vi "Engine-DI-Host.vi"() -> ()   [LabVIEW 2016]
uses:
  <vilib>/addons/Software Calibration Management/XControls/TBL2D.xctl
  <vilib>/Utility/miscctls.llb/LVRowAndColumnTypeDef.ctl
panel:
  in  "_Refresh PW Table":bool
  in  "_Hidden":enum32{"Page 1"}(tab)
  in  "InjQtys_Man":sgl[][](array[numeric]) caption="[]"
  in  "InjSplits":sgl[][](array[numeric]) caption="[]"
  out "CylFuelQtys":sgl[](array[numeric]) caption="[mm3/cycle/cyl]"
  in  "CylSplits":sgl[](array[numeric]) caption="[%]"
  out "InjQtys":sgl[][](array[numeric]) caption="[]"
  in  "_Refresh Table":bool
  out "Channels|Names":string[](array[string])
  out "Pulsewidths":sgl[][](array[numeric]) caption="[]"
  in  "_Bank Selection":T1(tab)
  out "TotalFuelQty":sgl caption="[mm3/cyc]"
  out "_Total Fueling Rate":sgl(graph) caption="[mm3/cyc]"
  in  "_Cylinder Fueling Control":i32(listbox) caption="DI Fueling Quantities"
  in  "InjQtys_ManE":bool caption="Mode Select"
  in  "_Cyl Split":sgl caption="Cylinder Split [%]"
  in  "_InjSplits":sgl[](array[numeric]) caption="Injection Splits [%]"
  in  "_InjQtys_Man":sgl[](array[numeric]) caption="Manual Injection Quantities [mm3/inj]"
  out "_Total Fueling Rate Indicator":sgl caption="[mm3/cyc]"
  in  "Enable":bool caption="Control Mode"
  in  "MinInjPW_A":sgl caption="[ms]"
  in  "InjFlowCal_A":cluster{"X":sgl[], "Y":sgl[], "Z":sgl[][]}(xcontrol) caption="[%|RPM|mm3/stroke]"
  in  "DI-A_RailPIndex":i32(ring) items=["None"=-1, "AI01"=0, "AI02"=1, "AI03"=2, "AI04"=3, "AI05"=4, "AI06"=5, "AI07"=6, "AI08"=7, "AI09"=8, "AI10"=9, "AI11"=10, "AI12"=11]
  out "DI-A_RailPSensor":T2 {"Value" format="%#_4p"}
  in  "MinInjPW_B":sgl caption="[ms]"
  in  "InjFlowCal_B":cluster{"X":sgl[], "Y":sgl[], "Z":sgl[][]}(xcontrol) caption="[%|RPM|mm3/stroke]"
  in  "DI-B_RailPIndex":i32(ring) items=["None"=-1, "AI01"=0, "AI02"=1, "AI03"=2, "AI04"=3, "AI05"=4, "AI06"=5, "AI07"=6, "AI08"=7, "AI09"=8, "AI10"=9, "AI11"=10, "AI12"=11]
  out "DI-B_RailPSensor":T2 {"Value" format="%#_4p"}
  in  "_Pulsewidths":i32(listbox) caption="DI Pulsewidths"
  # "DI Control and Calibration"
  # "Total DI Fueling Rate"
  # "RailP Sensor"
  # "Value"
  # "Units"
  # "RailP Sensor"
  # "Value"
  # "Units"
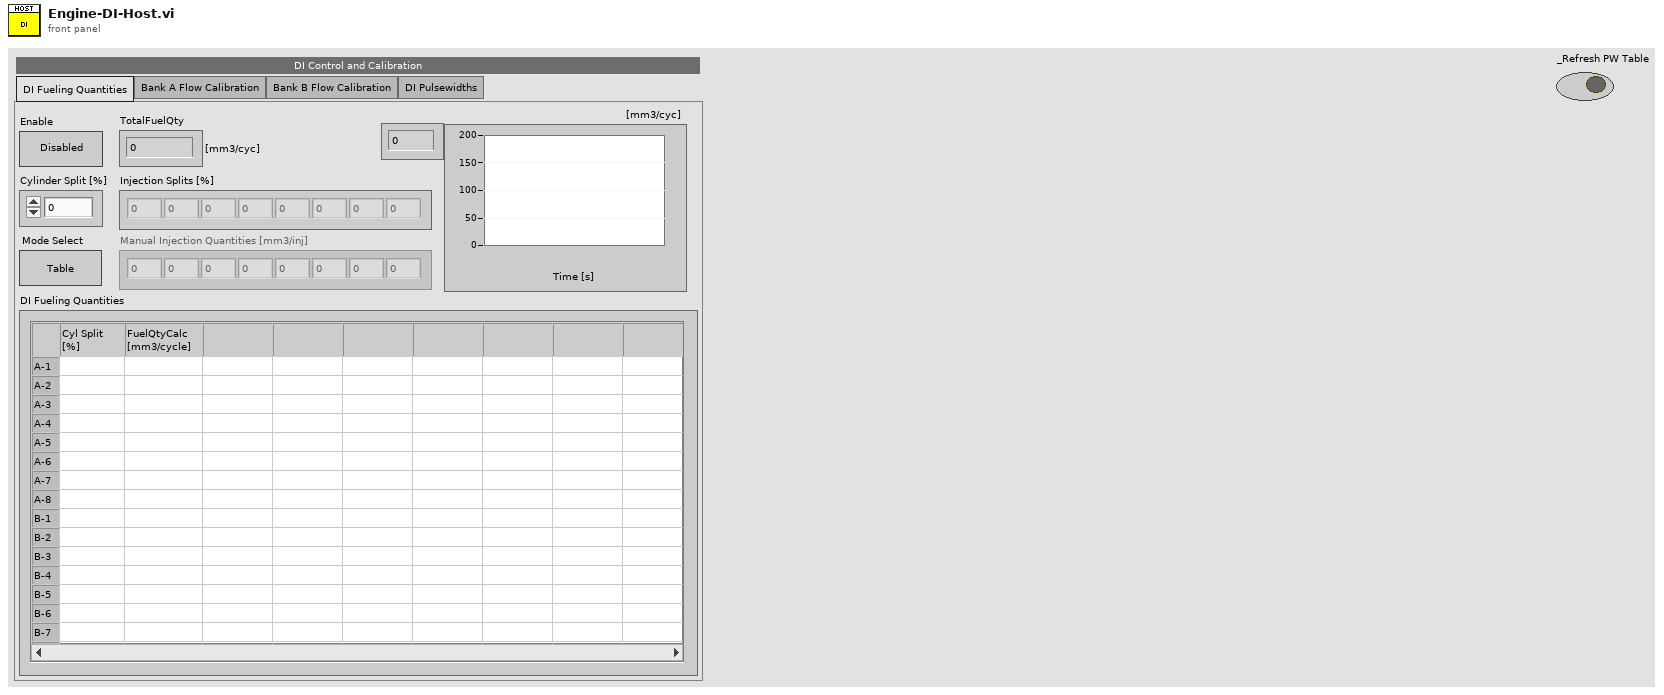
[diagram p1: front panel]
types:
  T1 = enum32{"DI Fueling Quantities", "Bank A Flow Calibration", "Bank B Flow Calibration", "DI Pulsewidths"}
  T2 = cluster{"Name":string, "Unit":string, "Value":sgl}
  T3 = typedef "LVRowAndColumnTypeDef.ctl" = cluster{"Row":i32, "Column":i32}
  T4 = enum8{"Enabled", "Disabled", "Disabled and Grayed Out"}
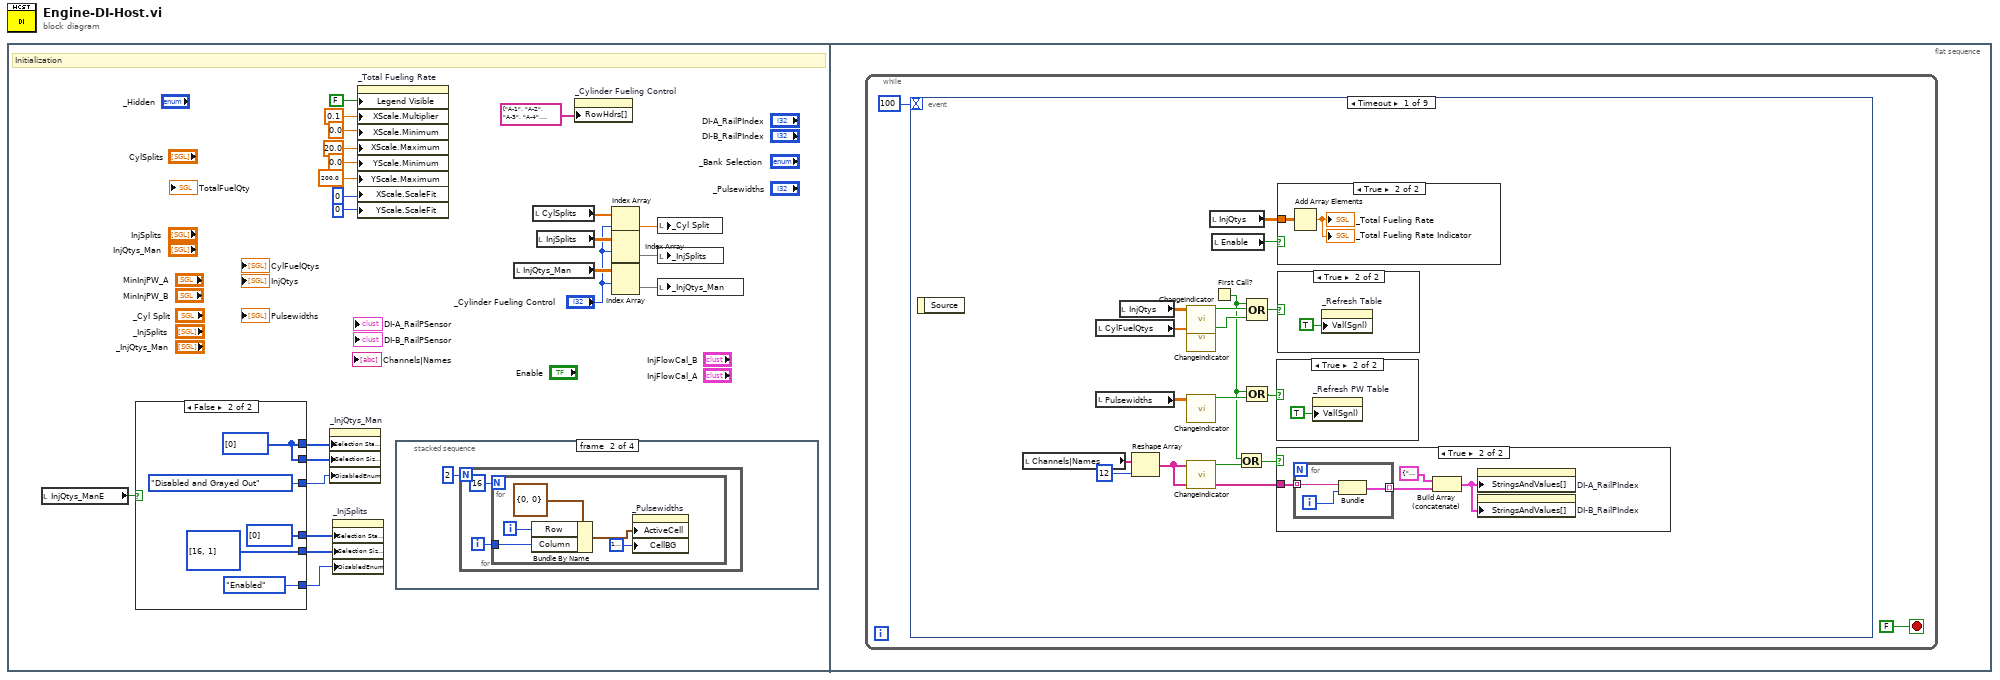
[diagram p0: block diagram]
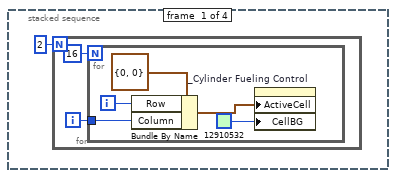
[diagram p2: hidden frame]
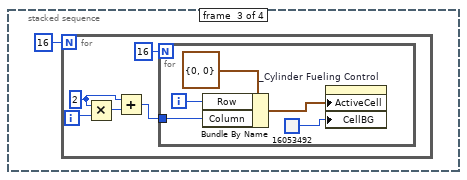
[diagram p3: hidden frame]
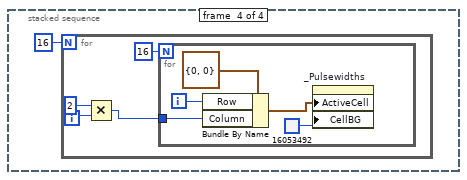
[diagram p4: hidden frame]
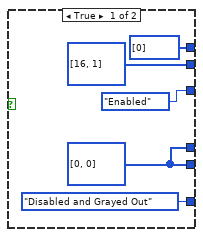
[diagram p5: hidden frame]
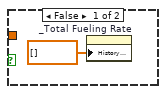
[diagram p9: hidden frame]
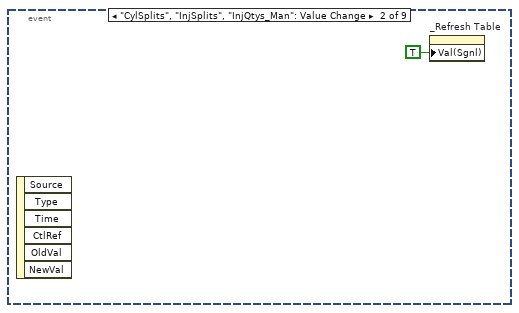
[diagram p10: hidden frame]
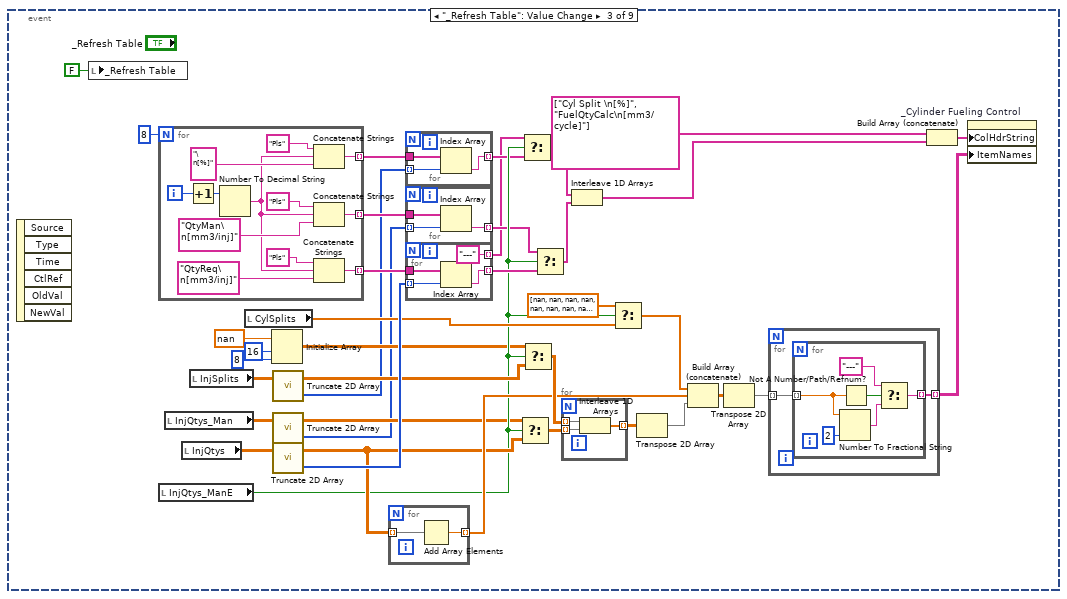
[diagram p11: hidden frame]
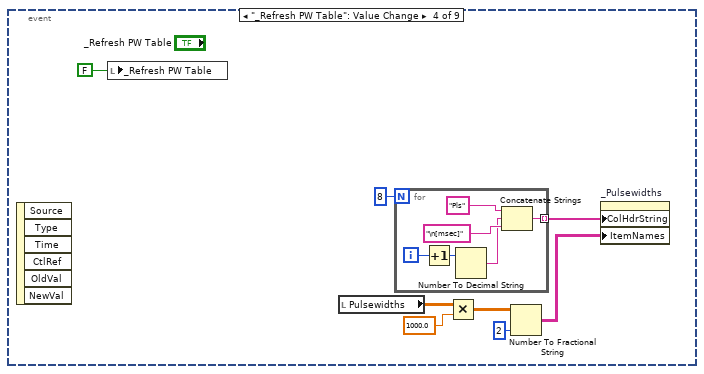
[diagram p12: hidden frame]
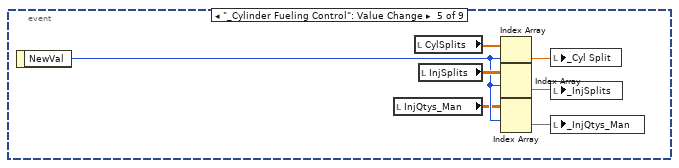
[diagram p13: hidden frame]
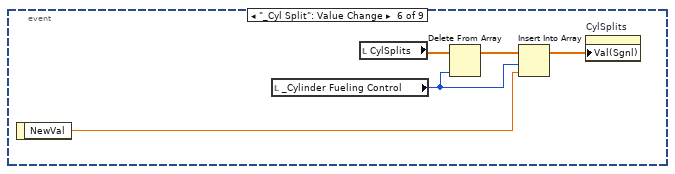
[diagram p14: hidden frame]
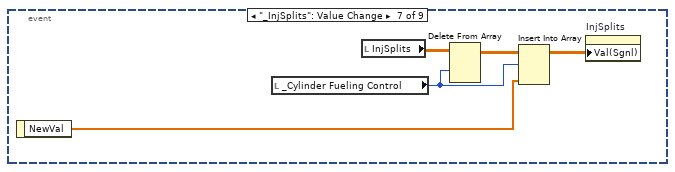
[diagram p15: hidden frame]
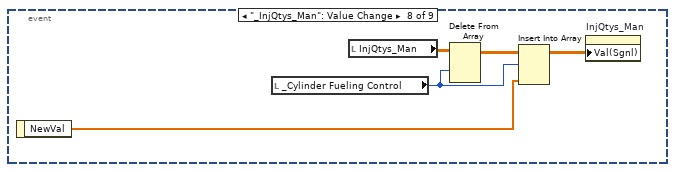
[diagram p16: hidden frame]
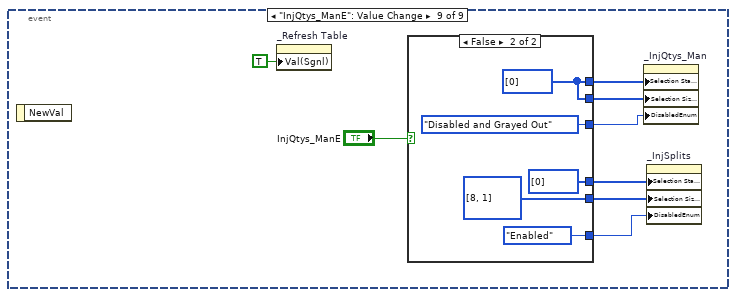
[diagram p17: hidden frame]
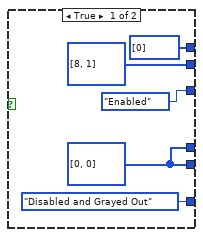
[diagram p18: hidden frame]
diagram:
  n1 = flat-sequence {
    frame #0 {
      # "Initialization"
      n2 = local read "InjQtys_ManE"() -> (w1:bool)
      n3 = case shown="False" w1 {
        tunnel: [u32[] [16, 1] ("Selection Start[]") w68] -> w7
        tunnel: [w63 u32[] [16, 1] ("Selection Start[]")] -> w6
        tunnel: [u32[] [0] ("Selection Size[]") w68] -> w5
        tunnel: [w63 u32[] [0] ("Selection Size[]")] -> w4
        tunnel: [T4."Enabled" ("Disabled") T4."Disabled and Grayed Out" ("Disabled")] -> w3
        tunnel: [T4."Disabled and Grayed Out" ("Disabled") T4."Enabled" ("Disabled")] -> w2
        frame True {
          w63 = u32[] [0, 0] ("Selection Start[]")
        }
        frame False {
          w68 = u32[] [0] ("Selection Size[]")
        }
      }
      n4 = property on="_InjQtys_Man" class="Arr (strict)"("Selection Start []"=w5, "Selection Size []"=w7, "DisabledEnum"=w3) -> ()  [unwired: 2 in, 2 out]
      n5 = property on="_InjSplits" class="Arr (strict)"("Selection Start []"=w4, "Selection Size []"=w6, "DisabledEnum"=w2) -> ()  [unwired: 2 in, 2 out]
      n6 = property on="_Total Fueling Rate" class="WFChart (strict)"("Legend Visible"=FALSE ("Legend:Visible"), "XScale.Multiplier"=0.1 ("X Scale.Range:Maximum"), "XScale.Minimum"=0.0 ("X Scale.Range:Minimum"), "XScale.Maximum"=20.0 ("X Scale.Range:Maximum"), "YScale.Minimum"=0.0 ("Y Scale.Range:Minimum"), "YScale.Maximum"=200.0 ("Y Scale.Range:Maximum"), "XScale.ScaleFit"=u8 0 ("X Scale.Scale Fit"), "YScale.ScaleFit"=u8 0 ("Y Scale.Scale Fit")) -> ()  [unwired: 2 in, 2 out]
      n7 = stacked-sequence {
        frame #0 {
          n8 = for {
            N: 2 -> [_]
            i -> [w25]
            n9 = for {
              N: 16 -> [_]
              tunnel: w25 -> [w27]
              i -> [w30]
              n10 = Bundle By Name(cluster=T3 {"Row"=0, "Column"=0} ("Active Cell:Active Cell"), "Row"=w30, "Column"=w27) -> (w29:T3)
              n11 = property on="_Cylinder Fueling Control" class="MCListbox (strict)"("ActiveCell"=w29, "CellBG"=u32 12910532) -> ()  [unwired: 2 in, 2 out]
            }
          }
        }
        frame #1 {
          n12 = for {
            N: 2 -> [_]
            i -> [w33]
            n13 = for {
              N: 16 -> [_]
              tunnel: w33 -> [w35]
              i -> [w38]
              n14 = Bundle By Name(cluster=T3 {"Row"=0, "Column"=0} ("Active Cell:Active Cell"), "Row"=w38, "Column"=w35) -> (w37:T3)
              n15 = property on="_Pulsewidths" class="MCListbox (strict)"("ActiveCell"=w37, "CellBG"=u32 16777226) -> ()  [unwired: 2 in, 2 out]
            }
          }
        }
        frame #2 {
          n16 = for {
            N: 16 -> [_]
            i -> [w44]
            w41 = 2
            n17 = Multiply(x=w41, y=w44) -> (x*y=w43:i32)
            n18 = Add(x=w41, y=w43) -> (x+y=w42:i32)
            n19 = for {
              N: 16 -> [_]
              tunnel: w42 -> [w47]
              i -> [w49]
              n20 = Bundle By Name(cluster=T3 {"Row"=0, "Column"=0} ("Active Cell:Active Cell"), "Row"=w49, "Column"=w47) -> (w48:T3)
              n21 = property on="_Cylinder Fueling Control" class="MCListbox (strict)"("ActiveCell"=w48, "CellBG"=u32 16053492) -> ()  [unwired: 2 in, 2 out]
            }
          }
        }
        frame #3 {
          n22 = for {
            N: 16 -> [_]
            i -> [w54]
            n23 = Multiply(x=2, y=w54) -> (x*y=w52:i32)
            n24 = for {
              N: 16 -> [_]
              tunnel: w52 -> [w57]
              i -> [w59]
              n25 = Bundle By Name(cluster=T3 {"Row"=0, "Column"=0} ("Active Cell:Active Cell"), "Row"=w59, "Column"=w57) -> (w58:T3)
              n26 = property on="_Pulsewidths" class="MCListbox (strict)"("ActiveCell"=w58, "CellBG"=u32 16053492) -> ()  [unwired: 2 in, 2 out]
            }
          }
        }
      }
      n27 = local read "InjQtys_Man"() -> (w22:sgl[][])
      n28 = local read "CylSplits"() -> (w18:sgl[])
      n29 = local read "InjSplits"() -> (w20:sgl[][])
      n30 = property on="_Cylinder Fueling Control" class="MCListbox (strict)"("RowHdrs[]"=string[] ["A-1", "A-2", "A-3", "A-4", "A-5", "A-6", "A-7", "A-8", "B-1", "B-2", "B-3", "B-4", "B-5", "B-6", "B-7", "B-8"] ("Row Header Strings[]")) -> ()  [unwired: 2 in, 2 out]
      n31 = Index Array(array=w18, index="_Cylinder Fueling Control") -> (element=w19:sgl)
      n32 = Index Array(array=w20, index (row)="_Cylinder Fueling Control") -> (element=w21:sgl[])  [unwired: 1 in]
      n33 = Index Array(array=w22, index (row)="_Cylinder Fueling Control") -> (element=w23:sgl[])  [unwired: 1 in]
      n34 = local write "_Cyl Split"(w19) -> ()
      n35 = local write "_InjSplits"(w21) -> ()
      n36 = local write "_InjQtys_Man"(w23) -> ()
    }
    frame #1 {
      n37 = while {
        stop <- FALSE stop-if-true
        n38 = event shown="[0] Timeout" {
          selector: _ -> [_ _ _ _ _ _ _ _ _]
          dyn-events: _ -> [_ _ _ _ _ _ _ _ _]
          timeout: 100 -> [_ _ _ _ _ _ _ _ _]
          event Timeout {
            n39 = event-data() -> ()  [unwired: 1 in, 1 out]
            n40 = local read "Channels|Names"() -> (w75:string[])
            n41 = local read "CylFuelQtys"() -> (w86:sgl[])
            n42 = local read "Pulsewidths"() -> (w81:sgl[][])
            n43 = local read "InjQtys"() -> (w85:sgl[][])
            n44 = Reshape Array(w75, 12 ("dimension size")) -> (w73:string[])
            n45 = call "ChangeIndicator.vi"("Input"=w85) -> ("Change"=w83:bool)  [unwired: 9 in]
            n46 = call "ChangeIndicator.vi"("Input"=w86) -> ("Change"=w84:bool)  [unwired: 9 in]
            n47 = call "ChangeIndicator.vi"("Input"=w81) -> ("Change"=w79:bool)  [unwired: 9 in]
            n48 = call "ChangeIndicator.vi"("Input"=w73) -> ("Change"=w77:bool)  [unwired: 9 in]
            n49 = local read "InjQtys"() -> (w87:sgl[][])
            n50 = First Call?() -> (First Call?: T/F=w78:bool)
            n51 = local read "Enable"() -> (w88:bool)
            n52 = Or(x=w78, y=w77) -> (x .or. y?=w76:bool)
            n53 = Compound Arithmetic op=OR(w78, w83, w84) -> (w82:bool)
            n54 = Compound Arithmetic op=OR(w78, w79) -> (w80:bool)
            n55 = case shown="True" w80 {
              frame False {
              }
              frame True {
                n56 = property on="_Refresh PW Table" class="Bool (strict)"("Val(Sgnl)"=TRUE ("Value (Signaling)")) -> ()  [unwired: 2 in, 2 out]
              }
            }
            n57 = case shown="True" w76 {
              tunnel: w73 -> [_ w92]
              frame False {
              }
              frame True {
                n58 = for {
                  tunnel: w92 -> [w95] mode=indexing
                  tunnel: [w93] -> w91 mode=indexing
                  i -> [w94]
                  n59 = Bundle("String"=w95, w94) -> (w93:cluster{"String":string, i32})  [unwired: 1 in]
                }
                n60 = Build Array (concatenate)(cluster{"String":string, i32} {"String"="None", -1} ("cluster"), w91) -> (w90:cluster{"String":string, i32}[])
                n61 = property on="DI-A_RailPIndex" class="Ring (strict)"("StringsAndValues[]"=w90) -> ()  [unwired: 2 in, 2 out]
                n62 = property on="DI-B_RailPIndex" class="Ring (strict)"("StringsAndValues[]"=w90) -> ()  [unwired: 2 in, 2 out]
              }
            }
            n63 = case shown="True" w88 {
              tunnel: w87 -> [_ w100]
              frame False {
                n64 = property on="_Total Fueling Rate" class="WFChart (strict)"("History Data"=sgl[] []) -> ()  [unwired: 2 in, 2 out]
              }
              frame True {
                n65 = Add Array Elements(numeric array=w100) -> (sum=→"_Total Fueling Rate" →"_Total Fueling Rate Indicator":sgl)
              }
            }
            n66 = case shown="True" w82 {
              frame False {
              }
              frame True {
                n67 = property on="_Refresh Table" class="Bool (strict)"("Val(Sgnl)"=TRUE ("Value (Signaling)")) -> ()  [unwired: 2 in, 2 out]
              }
            }
          }
          event "CylSplits", "InjSplits", "InjQtys_Man": Value Change {
            n68 = event-data() -> ()  [unwired: 1 in, 6 out]
            n69 = property on="_Refresh Table" class="Bool (strict)"("Val(Sgnl)"=TRUE ("Value (Signaling)")) -> ()  [unwired: 2 in, 2 out]
          }
          event "_Refresh Table": Value Change {
            n70 = event-data() -> ()  [unwired: 1 in, 6 out]
            n71 = local write "_Refresh Table"(FALSE ("_Refresh Table")) -> ()
            n72 = for {
              N: 8 -> [_]
              tunnel: [w172] -> w138 mode=indexing
              tunnel: [w168] -> w137 mode=indexing
              tunnel: [w164] -> w139 mode=indexing
              i -> [w175]
              n73 = Increment(x=w175) -> (x+1=w174:i32)
              n74 = Number To Decimal String(number=w174) -> (decimal integer string=w166:string)  [unwired: 1 in]
              n75 = Concatenate Strings("Pls", w166, "\n[%]") -> (w168:string)
              n76 = Concatenate Strings("Pls", w166, "QtyMan\n[mm3/inj]") -> (w172:string)
              n77 = Concatenate Strings("Pls", w166, "QtyReq\n[mm3/inj]") -> (w164:string)
            }
            n78 = local read "InjQtys_ManE"() -> (w109:bool)
            n79 = local read "InjQtys_Man"() -> (w130:sgl[][])
            n80 = local read "InjQtys"() -> (w129:sgl[][])
            n81 = local read "InjSplits"() -> (w131:sgl[][])
            n82 = local read "CylSplits"() -> (w127:sgl[])
            n83 = Initialize Array(sgl nan ("Numeric"), 16 ("dimension size"), 8 ("dimension size")) -> (w107:sgl[][])
            n84 = call "Truncate 2D Array.vi"("2D Array"=w131) -> ("Header Index"=w104:i32[], "Truncated 2D Array"=w136:sgl[][])  [unwired: 1 in]
            n85 = call "Truncate 2D Array.vi"("2D Array"=w130) -> ("Header Index"=w103:i32[], "Truncated 2D Array"=w108:sgl[][])  [unwired: 1 in]
            n86 = call "Truncate 2D Array.vi"("2D Array"=w129) -> ("Header Index"=w140:i32[], "Truncated 2D Array"=w113:sgl[][])  [unwired: 1 in]
            n87 = for {
              tunnel: w113 -> [w142] mode=indexing
              tunnel: [w141] -> w117 mode=indexing
              n88 = Add Array Elements(numeric array=w142) -> (sum=w141:sgl)
            }
            n89 = for {
              tunnel: w137 -> [w163]
              tunnel: w104 -> [w162] mode=indexing
              tunnel: [w161] -> w105 mode=indexing
              # "i"
              n90 = Index Array(array=w163, index=w162) -> (element=w161:string)
            }
            n91 = for {
              tunnel: w138 -> [w160]
              tunnel: w103 -> [w159] mode=indexing
              tunnel: [w158] -> w106 mode=indexing
              # "i"
              n92 = Index Array(array=w160, index=w159) -> (element=w158:string)
            }
            n93 = for {
              tunnel: w139 -> [w157]
              tunnel: w140 -> [w156] mode=indexing
              tunnel: [w155] -> w111 mode=indexing
              tunnel: ["---"] -> w102 mode=indexing
              # "i"
              n94 = Index Array(array=w157, index=w156) -> (element=w155:string)
            }
            n95 = Select(t=w108, s=w109, f=w113) -> (s? t:f=w112:sgl[][])
            n96 = Select(t=w102, s=w109, f=w105) -> (s? t:f=w120:string[])
            n97 = Select(t=w107, s=w109, f=w136) -> (s? t:f=w123:sgl[][])
            n98 = Select(t=w106, s=w109, f=w111) -> (s? t:f=w110:string[])
            n99 = for {
              tunnel: w123 -> [w145] mode=indexing
              tunnel: [w144] -> w122 mode=indexing
              tunnel: w112 -> [w143] mode=indexing
              n100 = Interleave 1D Arrays(w145, w143) -> (w144:sgl[])
            }
            n101 = Interleave 1D Arrays(w120, w110) -> (w119:string[])
            n102 = Select(t=sgl[] [nan, nan, nan, nan, nan, nan, nan, nan, nan, nan, nan, nan, nan, nan, nan, nan], s=w109, f=w127) -> (s? t:f=w126:sgl[])
            n103 = Transpose 2D Array(2D array=w122) -> (transposed array=w121:sgl[][])
            n104 = Build Array (concatenate)(w126, w117, w121) -> (w135:sgl[][])
            n105 = Transpose 2D Array(2D array=w135) -> (transposed array=w124:sgl[][])
            n106 = for {
              tunnel: w124 -> [w147] mode=indexing
              tunnel: [w146] -> w125 mode=indexing
              n107 = for {
                tunnel: w147 -> [w150] mode=indexing
                tunnel: [w148] -> w146 mode=indexing
                n108 = Number To Fractional String(number=w150, precision (6)=i16 2) -> (F-format string=w149:string)  [unwired: 2 in]
                n109 = Not A Number/Path/Refnum?(number/path/refnum=w150) -> (NaN/Path/Refnum?=w153:bool)
                n110 = Select(t="---", s=w153, f=w149) -> (s? t:f=w148:string)
              }
            }
            n111 = Build Array (concatenate)(string[] ["Cyl Split \n[%]", "FuelQtyCalc\n[mm3/cycle]"] ("Column Header Strings[]"), w119) -> (w134:string[])
            n112 = property on="_Cylinder Fueling Control" class="MCListbox (strict)"("ColHdrString"=w134, "ItemNames"=w125) -> ()  [unwired: 2 in, 2 out]
          }
          event "_Refresh PW Table": Value Change {
            n113 = event-data() -> ()  [unwired: 1 in, 6 out]
            n114 = local write "_Refresh PW Table"(FALSE ("_Refresh Table")) -> ()
            n115 = local read "Pulsewidths"() -> (w177:sgl[][])
            n116 = for {
              N: 8 -> [_]
              tunnel: [w185] -> w179 mode=indexing
              i -> [w189]
              n117 = Increment(x=w189) -> (x+1=w188:i32)
              n118 = Number To Decimal String(number=w188) -> (decimal integer string=w184:string)  [unwired: 1 in]
              n119 = Concatenate Strings("Pls", w184, "\n[msec]") -> (w185:string)
            }
            n120 = Multiply(x=w177, y=sgl 1000.0) -> (x*y=w178:sgl[][])
            n121 = Number To Fractional String(number=w178, precision (6)=i16 2) -> (F-format string=w180:string[][])  [unwired: 2 in]
            n122 = property on="_Pulsewidths" class="MCListbox (strict)"("ColHdrString"=w179, "ItemNames"=w180) -> ()  [unwired: 2 in, 2 out]
          }
          event "_Cylinder Fueling Control": Value Change {
            n123 = event-data() -> ("NewVal"=w192:i32)  [unwired: 1 in]
            n124 = local read "InjQtys_Man"() -> (w191:sgl[][])
            n125 = local read "CylSplits"() -> (w196:sgl[])
            n126 = local read "InjSplits"() -> (w194:sgl[][])
            n127 = Index Array(array=w196, index=w192) -> (element=w195:sgl)
            n128 = Index Array(array=w194, index (row)=w192) -> (element=w193:sgl[])  [unwired: 1 in]
            n129 = Index Array(array=w191, index (row)=w192) -> (element=w190:sgl[])  [unwired: 1 in]
            n130 = local write "_Cyl Split"(w195) -> ()
            n131 = local write "_InjSplits"(w193) -> ()
            n132 = local write "_InjQtys_Man"(w190) -> ()
          }
          event "_Cyl Split": Value Change {
            n133 = event-data() -> ("NewVal"=w197:sgl)  [unwired: 1 in]
            n134 = local read "_Cylinder Fueling Control"() -> (w201:i32)
            n135 = local read "CylSplits"() -> (w200:sgl[])
            n136 = Delete From Array(array=w200, index=w201) -> (array with subset deleted=w198:sgl[])  [unwired: 1 in, 1 out]
            n137 = Insert Into Array(array=w198, index=w201, new element=w197) -> (w199:sgl[])
            n138 = property on="CylSplits" class="Arr (strict)"("Val(Sgnl)"=w199) -> ()  [unwired: 2 in, 2 out]
          }
          event "_InjSplits": Value Change {
            n139 = event-data() -> ("NewVal"=w202:sgl[])  [unwired: 1 in]
            n140 = local read "_Cylinder Fueling Control"() -> (w206:i32)
            n141 = local read "InjSplits"() -> (w205:sgl[][])
            n142 = Delete From Array(array=w205, index (row)=w206) -> (array with subset deleted=w203:sgl[][])  [unwired: 2 in, 1 out]
            n143 = Insert Into Array(array=w203, index (row)=w206, new element=w202) -> (w204:sgl[][])  [unwired: 1 in]
            n144 = property on="InjSplits" class="Arr (strict)"("Val(Sgnl)"=w204) -> ()  [unwired: 2 in, 2 out]
          }
          event "_InjQtys_Man": Value Change {
            n145 = event-data() -> ("NewVal"=w207:sgl[])  [unwired: 1 in]
            n146 = local read "_Cylinder Fueling Control"() -> (w211:i32)
            n147 = local read "InjQtys_Man"() -> (w210:sgl[][])
            n148 = Delete From Array(array=w210, index (row)=w211) -> (array with subset deleted=w208:sgl[][])  [unwired: 2 in, 1 out]
            n149 = Insert Into Array(array=w208, index (row)=w211, new element=w207) -> (w209:sgl[][])  [unwired: 1 in]
            n150 = property on="InjQtys_Man" class="Arr (strict)"("Val(Sgnl)"=w209) -> ()  [unwired: 2 in, 2 out]
          }
          event "InjQtys_ManE": Value Change {
            n151 = event-data() -> ()  [unwired: 1 in, 1 out]
            n152 = property on="_Refresh Table" class="Bool (strict)"("Val(Sgnl)"=TRUE ("Value (Signaling)")) -> ()  [unwired: 2 in, 2 out]
            n153 = case shown="False" "InjQtys_ManE" {
              tunnel: [u32[] [8, 1] ("Selection Start[]") w227] -> w219
              tunnel: [w222 u32[] [8, 1] ("Selection Start[]")] -> w218
              tunnel: [u32[] [0] ("Selection Size[]") w227] -> w216
              tunnel: [w222 u32[] [0] ("Selection Size[]")] -> w215
              tunnel: [T4."Enabled" ("Disabled") T4."Disabled and Grayed Out" ("Disabled")] -> w214
              tunnel: [T4."Disabled and Grayed Out" ("Disabled") T4."Enabled" ("Disabled")] -> w213
              frame True {
                w222 = u32[] [0, 0] ("Selection Start[]")
              }
              frame False {
                w227 = u32[] [0] ("Selection Size[]")
              }
            }
            n154 = property on="_InjQtys_Man" class="Arr (strict)"("Selection Start []"=w216, "Selection Size []"=w219, "DisabledEnum"=w214) -> ()  [unwired: 2 in, 2 out]
            n155 = property on="_InjSplits" class="Arr (strict)"("Selection Start []"=w215, "Selection Size []"=w218, "DisabledEnum"=w213) -> ()  [unwired: 2 in, 2 out]
          }
        }
      }
    }
  }
